vi "CycleHistoryTable.vi"(5 "Low Level Tries":u8=5, 7 "Error In":errorcluster, 8 "Cycle History ERD":T1={"ERD Number"=57629, "Data Type"=enum."string"} {"ERD Number" format="%.0x"}, 9 "GEA Inputs":T3={"Source"=228, "Destination"=36} {"Destination" format="%.0x"; "Source" format="%.0x"}, 10 "GEA2 Reference In":refnum<k24>) -> (0 "Error Out":errorcluster, 1 "String Array Out":string[](array[string]), 2 "Cluster Data Out":T4, 3 "GEA2 Reference Out":refnum<k24>)   [LabVIEW 2016]
uses:
  type defs/CycleHistoryControl.ctl
  Q:/Common/DLLs/GEA3/GeaCommunication.dll
  Common/DLLs/GEA3/GeaCommunication.dll
  Common/LabVIEW GEA2 Toolkit/LabVIEW_GEA2_Toolkit.lvlibp/type defs/Source_Destination.ctl
  Common/LabVIEW GEA2 Toolkit/LabVIEW_GEA2_Toolkit.lvlibp/type defs/ERD Read Data In.ctl
  Common/LabVIEW GEA2 Toolkit/LabVIEW_GEA2_Toolkit.lvlibp/type defs/Data Type.ctl
  Common/LabVIEW GEA2 Toolkit/LabVIEW_GEA2_Toolkit.lvlibp
panel:
  # "**Note: Two unused bytes at end**"
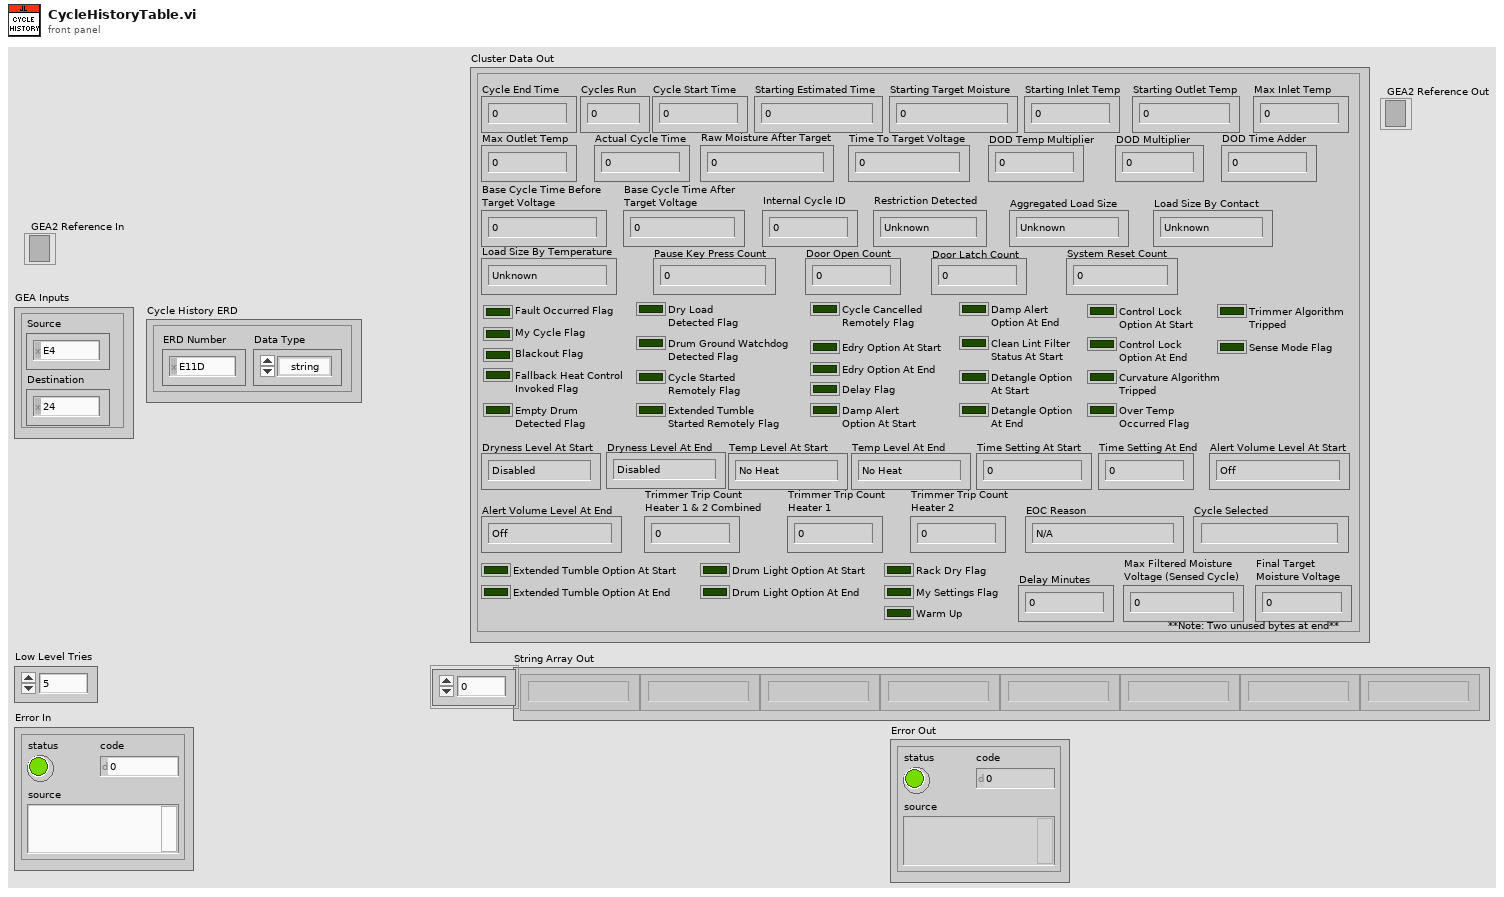
[diagram p1: front panel]
types:
  T1 = typedef "LabVIEW_GEA2_Toolkit.lvlibp/ERD Read Data In.ctl" = cluster{"ERD Number":u16, "Data Type":T2}
  T2 = typedef "LabVIEW_GEA2_Toolkit.lvlibp/Data Type.ctl" = enum16{"string", "boolean", "uint8_t", "uint16_t", "uint32_t", "uint64_t", "int8_t", "int16_t", "int32_t", "int64_t"}
  T3 = typedef "LabVIEW_GEA2_Toolkit.lvlibp/Source_Destination.ctl" = cluster{"Source":u8, "Destination":u8}
  T4 = typedef "CycleHistoryControl.ctl" = cluster{"Cycle End Time":u32, "Cycles Run":u32, "Cycle Start Time":u32, "Starting Estimated Time":u16, "Starting Target Moisture":u16, "Starting Inlet Temp":u16, "Starting Outlet Temp":u16, "Max Inlet Temp":u16, "Max Outlet Temp":u16, "Dryness Level At Start":enum8{"Disabled", "Damp", "Less Dry", "Dry", "More Dry", "Extra Dry"}, "Dryness Level At End":enum8{"Disabled", "Damp", "Less Dry", "Dry", "More Dry", "Extra Dry"}, "Temp Level At Start":enum8{"No Heat", "Extra Low", "Low", "Medium", "High"}, "Temp Level At End":enum8{"No Heat", "Extra Low", "Low", "Medium", "High"}, "Time Setting At Start":u8, "Time Setting At End":u8, "Trimmer Trip Count\nHeater 1 & 2 Combined":u8, "Trimmer Trip Count\nHeater 1":u8, "Trimmer Trip Count\nHeater 2":u8, "EOC Reason":enum16{"N/A", "Empty Drum", "Dry Load", "Cool Down Paused", "Extended Tumble Paused", "Knob Change", "Power Key", "Normal", "Event Sequence Communication Issue"}, "Cycle Selected":string, "Actual Cycle Time":u16, "Raw Moisture After Target":u16, "Time To Target Voltage":u16, "DOD Temp Multiplier":u16, "DOD Multiplier":u8, "DOD Time Adder":u8, "Base Cycle Time Before\nTarget Voltage":u8, "Base Cycle Time After\nTarget Voltage":u8, "Internal Cycle ID":u8, "Restriction Detected":enum8{"Unknown", "Small", "Large"}, "Aggregated Load Size":enum8{"Unknown", "Small", "Large"}, "Load Size By Contact":enum8{"Unknown", "Small", "Large"}, "Load Size By Temperature":enum8{"Unknown", "Small", "Large"}, "Pause Key Press Count":u8, "Door Open Count":u8, "Door Latch Count":u8, "System Reset Count":u8, "Fault Occurred Flag":bool, "My Cycle Flag":bool, "Blackout Flag":bool, "Fallback Heat Control\nInvoked Flag":bool, "Empty Drum \nDetected Flag":bool, "Dry Load \nDetected Flag":bool, "Drum Ground Watchdog\nDetected Flag":bool, "Cycle Started\nRemotely Flag":bool, "Extended Tumble\nStarted Remotely Flag":bool, "Cycle Cancelled\nRemotely Flag":bool, "Edry Option At Start":bool, "Edry Option At End":bool, "Delay Flag":bool, "Damp Alert\nOption At Start":bool, "Damp Alert\nOption At End":bool, "Clean Lint Filter\nStatus At Start":bool, "Detangle Option\nAt Start":bool, "Detangle Option\nAt End":bool, "Control Lock\nOption At Start":bool, "Control Lock\nOption At End":bool, "Curvature Algorithm\nTripped":bool, "Over Temp\nOccurred Flag":bool, "Trimmer Algorithm\nTripped":bool, "Sense Mode Flag":bool, "Extended Tumble Option At Start":bool, "Extended Tumble Option At End":bool, "Drum Light Option At Start":bool, "Drum Light Option At End":bool, "Rack Dry Flag":bool, "My Settings Flag":bool, "Warm Up":bool, "Delay Minutes":u16, "Alert Volume Level At Start":enum8{"Off", "Low", "Medium", "High"}, "Alert Volume Level At End":enum8{"Off", "Low", "Medium", "High"}, "Max Filtered Moisture\nVoltage (Sensed Cycle)":u16, "Final Target\nMoisture Voltage":u16}
  T5 = enum8{"Disabled", "Damp", "Less Dry", "Dry", "More Dry", "Extra Dry"}
  T6 = enum8{"No Heat", "Extra Low", "Low", "Medium", "High"}
  T7 = enum16{"N/A", "Empty Drum", "Dry Load", "Cool Down Paused", "Extended Tumble Paused", "Knob Change", "Power Key", "Normal", "Event Sequence Communication Issue"}
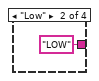
[diagram p4: hidden frame]
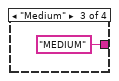
[diagram p5: hidden frame]
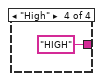
[diagram p6: hidden frame]
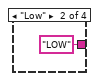
[diagram p7: hidden frame]
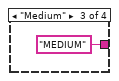
[diagram p8: hidden frame]
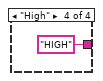
[diagram p9: hidden frame]
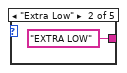
[diagram p10: hidden frame]
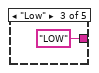
[diagram p11: hidden frame]
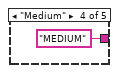
[diagram p12: hidden frame]
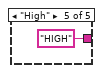
[diagram p13: hidden frame]
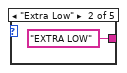
[diagram p14: hidden frame]
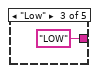
[diagram p15: hidden frame]
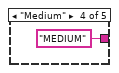
[diagram p16: hidden frame]
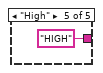
[diagram p17: hidden frame]
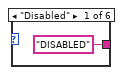
[diagram p18: hidden frame]
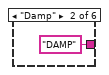
[diagram p19: hidden frame]
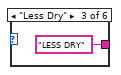
[diagram p20: hidden frame]
diagram:
  w24 = 3 ("offset (0)")
  w199 = 0 ("offset (0)")
  # "Final Target\nMoisture Voltage"
  # "Max Filtered Mosture\nDuring a Sensed Cycle"
  # "Take in a 1D array of ERD data\nfrom another VI & index that array\nto pull out the data. \n\nWe will parse this data in the next step..."
  # "Build a 1D array of strings \ncontaining all clustered data"
  # "Unbundle clustered data,\nthen format into string to\nobtain all clustered data as \none singlular string"
  # "Output clustered data\n& move to unbundle\ndata to format into \none string"
  # "Parse the data byte by byte...\nadd 3 each time since  each byte's\nlength is 2 numbers + 1 space character.\n\nThis number we are adding takes a subset\nof the data string to know which byte\nlocation we want to pull data from each time."
  # "Can try to use 'format into string' VI to\nsimplify this part, but should work as is."
  # "Alert Volume Level At End"
  # "Alert Volume Level At Start"
  # "Warm Up"
  # "Delay Minutes"
  # "=====CLUSTER ARRAY====="
  # "=====STRING ARRAY====="
  # "My Settings Flag"
  # "Rack Dry Flag"
  # "Drum Light Option At End"
  # "Drum Light Option At Start"
  # "Extended Tumble Option At End"
  # "Extended Tumble Option At Start"
  # "Boolean Byte #4"
  # "Cycle Selected"
  # "EOC Reason"
  # "Trimmer Trip Count Heater 2"
  # "Trimmer Trip Count Heater 1"
  # "Trimmer Trip Count\n Heater 1 & 2 Combined"
  # "Time Setting At End"
  # "Time Setting At Start"
  # "Temp Level At End"
  # "Temp Level At Start"
  # "Dryness Level At End"
  # "Dryness Level At Start"
  # "Sense Mode Flag"
  # "Trimmer Algorithm Tripped"
  # "Over Temperature Occurred Flag"
  # "Curvature Algorithm Tripped"
  # "Control Lock Option At End"
  # "Control Lock Option At Start"
  # "Detangle Option At End"
  # "Detangle Option At Start"
  # "Boolean Byte #3"
  # "Clean Lint Filter Status At Start"
  # "Damp Alert Option At End"
  # "Damp Alert Option At Start"
  # "Edry Option At End"
  # "Edry Option At Start"
  # "Cycle Cancelled Remotely Flag"
  # "Extended Tumble Started Remotely Flag"
  # "Cycle Started Remotely Flag"
  # "Boolean Byte #2"
  # "Drum Ground Watchdog Detected Flag"
  # "Dry Load Detected Flag"
  # "Empty Drum Detected Flag"
  # "Fallback Heat Control Invoked Flag"
  # "Blackout Flag"
  # "My Cycle Flag"
  # "Delay Flag"
  # "Fault Occurred Flag"
  # "Boolean Byte #1"
  # "Door Latch Count"
  # "System Reset Count"
  # "Door Open Count"
  # "Pause Key Press Count"
  # "Load Size By Temperature"
  # "Load Size By Contact"
  # "Aggregated Load Size"
  # "Restriction Detected"
  # "Internal Cycle ID"
  # "Base Cycle Time After\nTarget Voltage"
  # "Base Cycle Time Before\nTarget Voltage"
  # "DOD Time Adder"
  # "DOD Multiplier"
  # "DOD Temp Multiplier"
  # "Time To Target Voltage"
  # "Raw Moisture After Target"
  # "Actual Cycle Time"
  # "Max Outlet Temp"
  # "Max Inlet Temp"
  # "Starting Outlet Temp"
  # "Starting Inlet Temp"
  # "Starting Target Moisture"
  # "Starting Estimated Time"
  # "Cycle Start Time"
  # "Cycles Run"
  # "Cycle End Time"
  n1 = Not A Number/Path/Refnum?(number/path/refnum="GEA2 Reference In") -> (NaN/Path/Refnum?=w15:bool)
  n2 = case shown="True" w15 {
    tunnel: "GEA Inputs" -> [_ w635]
    tunnel: "Error In" -> [w630 w634]
    tunnel: [w630 w633] -> w8
    tunnel: [w629 w632] -> w13
    tunnel: "GEA2 Reference In" -> [w629 _]
    frame False {
    }
    frame True {
      n3 = Unbundle By Name(w635) -> ("Source"=w631:u8)
      n4 = call "GEA2 Initialize.vi"("Source Address"=w631, "error in"=w634) -> ("GEA2 Reference Out"=w632:refnum<k24>, "error out"=w633:errorcluster)  [unwired: 11 in, 1 out]
    }
  }
  n5 = Build Array("Cycle History ERD") -> (w4:T1[])
  n6 = call "GEA2 Read ERD.vi"("GEA2 Reference In"=w13, "GEA Inputs"="GEA Inputs", "Read ERD List"=w4, "Error In"=w8, "Low Level Tries"="Low Level Tries") -> ("GEA2 Reference Out"=w11:refnum<k24>, "Raw Data Out"=w9:string, "Error Out"=w10:errorcluster)  [unwired: 7 in, 1 out]
  n7 = case shown="True" w15 {
    tunnel: [w636 w640] -> w16
    tunnel: [w637 _] -> w14
    tunnel: w11 -> [w637 w638]
    tunnel: w10 -> [w636 w639]
    frame False {
    }
    frame True {
      n8 = call "GEA2 Stop.vi"("GEA2 Reference In"=w638, "Error In"=w639) -> ("Error Out"=w640:errorcluster)  [unwired: 13 in]
    }
  }
  "Error Out" <- w16
  "GEA2 Reference Out" <- w14
  n9 = String Subset(string=w9, offset (0)=28) -> (substring=w2:string)  [unwired: 1 in]
  n10 = call "String Remove All Spaces.vi"("Input String"=w2) -> ("Spaces Removed"=w1:string)  [unwired: 13 in, 1 out]
  n11 = Add(x=w199, y=w24) -> (x+y=w198:i32)
  n12 = Add(x=w198, y=w24) -> (x+y=w197:i32)
  n13 = Add(x=w197, y=w24) -> (x+y=w196:i32)
  n14 = Add(x=w196, y=w24) -> (x+y=w195:i32)
  n15 = Add(x=w195, y=w24) -> (x+y=w194:i32)
  n16 = Add(x=w194, y=w24) -> (x+y=w193:i32)
  n17 = Add(x=w193, y=w24) -> (x+y=w192:i32)
  n18 = Add(x=w192, y=w24) -> (x+y=w191:i32)
  n19 = Add(x=w191, y=w24) -> (x+y=w190:i32)
  n20 = Add(x=w190, y=w24) -> (x+y=w189:i32)
  n21 = Add(x=w189, y=w24) -> (x+y=w188:i32)
  n22 = Add(x=w188, y=w24) -> (x+y=w187:i32)
  n23 = Add(x=w187, y=w24) -> (x+y=w186:i32)
  n24 = Add(x=w186, y=w24) -> (x+y=w185:i32)
  n25 = Add(x=w185, y=w24) -> (x+y=w184:i32)
  n26 = Add(x=w184, y=w24) -> (x+y=w183:i32)
  n27 = Add(x=w183, y=w24) -> (x+y=w182:i32)
  n28 = Add(x=w182, y=w24) -> (x+y=w181:i32)
  n29 = Add(x=w181, y=w24) -> (x+y=w180:i32)
  n30 = Add(x=w180, y=w24) -> (x+y=w179:i32)
  n31 = Add(x=w179, y=w24) -> (x+y=w178:i32)
  n32 = Add(x=w178, y=w24) -> (x+y=w177:i32)
  n33 = Add(x=w177, y=w24) -> (x+y=w176:i32)
  n34 = Add(x=w176, y=w24) -> (x+y=w175:i32)
  n35 = Add(x=w175, y=w24) -> (x+y=w174:i32)
  n36 = Add(x=w174, y=w24) -> (x+y=w173:i32)
  n37 = Add(x=w173, y=w24) -> (x+y=w172:i32)
  n38 = Add(x=w172, y=w24) -> (x+y=w171:i32)
  n39 = Add(x=w171, y=w24) -> (x+y=w170:i32)
  n40 = Add(x=w170, y=w24) -> (x+y=w169:i32)
  n41 = Add(x=w169, y=w24) -> (x+y=w160:i32)
  n42 = Add(x=w160, y=w24) -> (x+y=w158:i32)
  n43 = Add(x=w158, y=w24) -> (x+y=w157:i32)
  n44 = Add(x=w157, y=w24) -> (x+y=w150:i32)
  n45 = Add(x=w150, y=w24) -> (x+y=w148:i32)
  n46 = Add(x=w148, y=w24) -> (x+y=w146:i32)
  n47 = Add(x=w146, y=w24) -> (x+y=w144:i32)
  n48 = Add(x=w144, y=w24) -> (x+y=w142:i32)
  n49 = Add(x=w142, y=w24) -> (x+y=w140:i32)
  n50 = Add(x=w140, y=w24) -> (x+y=w137:i32)
  n51 = Add(x=w137, y=w24) -> (x+y=w136:i32)
  n52 = Add(x=w136, y=w24) -> (x+y=w134:i32)
  n53 = Add(x=w134, y=w24) -> (x+y=w132:i32)
  n54 = Add(x=w132, y=w24) -> (x+y=w130:i32)
  n55 = Add(x=w130, y=w24) -> (x+y=w128:i32)
  n56 = Add(x=w128, y=w24) -> (x+y=w126:i32)
  n57 = Add(x=w126, y=w24) -> (x+y=w124:i32)
  n58 = Add(x=w124, y=w24) -> (x+y=w122:i32)
  n59 = Add(x=w122, y=w24) -> (x+y=w120:i32)
  n60 = Add(x=w120, y=w24) -> (x+y=w118:i32)
  n61 = Add(x=w118, y=w24) -> (x+y=w116:i32)
  n62 = Add(x=w116, y=w24) -> (x+y=w114:i32)
  n63 = Add(x=w114, y=w24) -> (x+y=w112:i32)
  n64 = Add(x=w112, y=w24) -> (x+y=w110:i32)
  n65 = Add(x=w110, y=w24) -> (x+y=w76:i32)
  n66 = Add(x=w76, y=w24) -> (x+y=w78:i32)
  n67 = Add(x=w78, y=w24) -> (x+y=w73:i32)
  n68 = Add(x=w73, y=w24) -> (x+y=w107:i32)
  n69 = Add(x=w107, y=w24) -> (x+y=w105:i32)
  n70 = Add(x=w105, y=w24) -> (x+y=w103:i32)
  n71 = Add(x=w103, y=w24) -> (x+y=w101:i32)
  n72 = Add(x=w101, y=w24) -> (x+y=w94:i32)
  n73 = Add(x=w94, y=w24) -> (x+y=w92:i32)
  n74 = Add(x=w92, y=w24) -> (x+y=w90:i32)
  n75 = Add(x=w90, y=w24) -> (x+y=w41:i32)
  n76 = Add(x=w41, y=w24) -> (x+y=w38:i32)
  n77 = Add(x=w38, y=w24) -> (x+y=w25:i32)
  n78 = Add(x=w25, y=w24) -> (x+y=w31:i32)
  n79 = Add(x=w31, y=w24) -> (x+y=w30:i32)
  n80 = String Subset(string=w1, offset (0)=w198, length (rest)=2 ("length (rest)")) -> (substring=w622:string)
  n81 = String Subset(string=w1, offset (0)=w194, length (rest)=2 ("length (rest)")) -> (substring=w613:string)
  n82 = String Subset(string=w1, offset (0)=w199, length (rest)=2 ("length (rest)")) -> (substring=w623:string)
  n83 = String Subset(string=w1, offset (0)=w195, length (rest)=2 ("length (rest)")) -> (substring=w614:string)
  n84 = String Subset(string=w1, offset (0)=w197, length (rest)=2 ("length (rest)")) -> (substring=w621:string)
  n85 = String Subset(string=w1, offset (0)=w193, length (rest)=2 ("length (rest)")) -> (substring=w612:string)
  n86 = String Subset(string=w1, offset (0)=w196, length (rest)=2 ("length (rest)")) -> (substring=w620:string)
  n87 = String Subset(string=w1, offset (0)=w192, length (rest)=2 ("length (rest)")) -> (substring=w611:string)
  n88 = String Subset(string=w1, offset (0)=w190, length (rest)=2 ("length (rest)")) -> (substring=w602:string)
  n89 = String Subset(string=w1, offset (0)=w184, length (rest)=2 ("length (rest)")) -> (substring=w589:string)
  n90 = String Subset(string=w1, offset (0)=w183, length (rest)=2 ("length (rest)")) -> (substring=w583:string)
  n91 = String Subset(string=w1, offset (0)=w191, length (rest)=2 ("length (rest)")) -> (substring=w603:string)
  n92 = String Subset(string=w1, offset (0)=w185, length (rest)=2 ("length (rest)")) -> (substring=w590:string)
  n93 = String Subset(string=w1, offset (0)=w182, length (rest)=2 ("length (rest)")) -> (substring=w582:string)
  n94 = String Subset(string=w1, offset (0)=w186, length (rest)=2 ("length (rest)")) -> (substring=w595:string)
  n95 = String Subset(string=w1, offset (0)=w181, length (rest)=2 ("length (rest)")) -> (substring=w576:string)
  n96 = String Subset(string=w1, offset (0)=w187, length (rest)=2 ("length (rest)")) -> (substring=w596:string)
  n97 = String Subset(string=w1, offset (0)=w180, length (rest)=2 ("length (rest)")) -> (substring=w575:string)
  n98 = String Subset(string=w1, offset (0)=w189, length (rest)=2 ("length (rest)")) -> (substring=w601:string)
  n99 = String Subset(string=w1, offset (0)=w188, length (rest)=2 ("length (rest)")) -> (substring=w600:string)
  n100 = String Subset(string=w1, offset (0)=w179, length (rest)=2 ("length (rest)")) -> (substring=w569:string)
  n101 = String Subset(string=w1, offset (0)=w178, length (rest)=2 ("length (rest)")) -> (substring=w568:string)
  n102 = String Subset(string=w1, offset (0)=w177, length (rest)=2 ("length (rest)")) -> (substring=w563:string)
  n103 = String Subset(string=w1, offset (0)=w176, length (rest)=2 ("length (rest)")) -> (substring=w562:string)
  n104 = String Subset(string=w1, offset (0)=w92, length (rest)=2 ("length (rest)")) -> (substring=w342:string)
  n105 = String Subset(string=w1, offset (0)=w175, length (rest)=2 ("length (rest)")) -> (substring=w555:string)
  n106 = String Subset(string=w1, offset (0)=w103, length (rest)=2 ("length (rest)")) -> (substring=w355:string)
  n107 = String Subset(string=w1, offset (0)=w94, length (rest)=2 ("length (rest)")) -> (substring=w346:string)
  n108 = String Subset(string=w1, offset (0)=w174, length (rest)=2 ("length (rest)")) -> (substring=w554:string)
  n109 = String Subset(string=w1, offset (0)=w76, length (rest)=2 ("length (rest)")) -> (substring=w362:string)
  n110 = String Subset(string=w1, offset (0)=w107, length (rest)=2 ("length (rest)")) -> (substring=w357:string)
  n111 = String Subset(string=w1, offset (0)=w105, length (rest)=2 ("length (rest)")) -> (substring=w356:string)
  n112 = String Subset(string=w1, offset (0)=w101, length (rest)=2 ("length (rest)")) -> (substring=w351:string)
  n113 = String Subset(string=w1, offset (0)=w173, length (rest)=2 ("length (rest)")) -> (substring=w549:string)
  n114 = String Subset(string=w1, offset (0)=w144, length (rest)=2 ("length (rest)")) -> (substring=w527:string)
  n115 = String Subset(string=w1, offset (0)=w110, length (rest)=2 ("length (rest)")) -> (substring=w363:string)
  n116 = String Subset(string=w1, offset (0)=w172, length (rest)=2 ("length (rest)")) -> (substring=w548:string)
  n117 = String Subset(string=w1, offset (0)=w146, length (rest)=2 ("length (rest)")) -> (substring=w529:string)
  n118 = String Subset(string=w1, offset (0)=w112, length (rest)=2 ("length (rest)")) -> (substring=w367:string)
  n119 = String Subset(string=w1, offset (0)=w142, length (rest)=2 ("length (rest)")) -> (substring=w523:string)
  n120 = String Subset(string=w1, offset (0)=w116, length (rest)=2 ("length (rest)")) -> (substring=w369:string)
  n121 = String Subset(string=w1, offset (0)=w114, length (rest)=2 ("length (rest)")) -> (substring=w368:string)
  n122 = String Subset(string=w1, offset (0)=w31, length (rest)=2 ("length (rest)")) -> (substring=w29:string)
  n123 = String Subset(string=w1, offset (0)=w148, length (rest)=2 ("length (rest)")) -> (substring=w154:string)
  n124 = String Subset(string=w1, offset (0)=w134, length (rest)=2 ("length (rest)")) -> (substring=w515:string)
  n125 = String Subset(string=w1, offset (0)=w118, length (rest)=2 ("length (rest)")) -> (substring=w371:string)
  n126 = String Subset(string=w1, offset (0)=w90, length (rest)=2 ("length (rest)")) -> (substring=w99:string)
  n127 = String Subset(string=w1, offset (0)=w41, length (rest)=2 ("length (rest)")) -> (substring=w98:string)
  n128 = String Subset(string=w1, offset (0)=w30, length (rest)=2 ("length (rest)")) -> (substring=w28:string)
  n129 = String Subset(string=w1, offset (0)=w171, length (rest)=2 ("length (rest)")) -> (substring=w541:string)
  n130 = String Subset(string=w1, offset (0)=w157, length (rest)=2 ("length (rest)")) -> (substring=w165:string)
  n131 = String Subset(string=w1, offset (0)=w170, length (rest)=2 ("length (rest)")) -> (substring=w540:string)
  n132 = String Subset(string=w1, offset (0)=w150, length (rest)=2 ("length (rest)")) -> (substring=w155:string)
  n133 = String Subset(string=w1, offset (0)=w132, length (rest)=2 ("length (rest)")) -> (substring=w512:string)
  n134 = String Subset(string=w1, offset (0)=w169, length (rest)=2 ("length (rest)")) -> (substring=w535:string)
  n135 = String Subset(string=w1, offset (0)=w158, length (rest)=2 ("length (rest)")) -> (substring=w166:string)
  n136 = String Subset(string=w1, offset (0)=w137, length (rest)=2 ("length (rest)")) -> (substring=w518:string)
  n137 = String Subset(string=w1, offset (0)=w136, length (rest)=2 ("length (rest)")) -> (substring=w516:string)
  n138 = String Subset(string=w1, offset (0)=w130, length (rest)=2 ("length (rest)")) -> (substring=w511:string)
  n139 = String Subset(string=w1, offset (0)=w120, length (rest)=2 ("length (rest)")) -> (substring=w430:string)
  n140 = String Subset(string=w1, offset (0)=w160, length (rest)=2 ("length (rest)")) -> (substring=w534:string)
  n141 = String Subset(string=w1, offset (0)=w128, length (rest)=2 ("length (rest)")) -> (substring=w510:string)
  n142 = String Subset(string=w1, offset (0)=w126, length (rest)=2 ("length (rest)")) -> (substring=w509:string)
  n143 = String Subset(string=w1, offset (0)=w140, length (rest)=2 ("length (rest)")) -> (substring=w520:string)
  n144 = String Subset(string=w1, offset (0)=w122, length (rest)=2 ("length (rest)")) -> (substring=w465:string)
  n145 = String Subset(string=w1, offset (0)=w124, length (rest)=2 ("length (rest)")) -> (substring=w500:string)
  n146 = String Subset(string=w1, offset (0)=w73, length (rest)=2 ("length (rest)")) -> (substring=w80:string)
  n147 = String Subset(string=w1, offset (0)=w38, length (rest)=2 ("length (rest)")) -> (substring=w37:string)
  n148 = String Subset(string=w1, offset (0)=w78, length (rest)=2 ("length (rest)")) -> (substring=w81:string)
  n149 = String Subset(string=w1, offset (0)=w25, length (rest)=2 ("length (rest)")) -> (substring=w36:string)
  n150 = Hexadecimal String To Number(string=w342) -> (number=w341:u32)  [unwired: 2 in, 1 out]
  n151 = Concatenate Strings(w623, w622, w621, w620) -> (w619:string)
  n152 = Concatenate Strings(w614, w613, w612, w611) -> (w610:string)
  n153 = Concatenate Strings(w590, w589) -> (w588:string)
  n154 = Concatenate Strings(w603, w602, w601, w600) -> (w599:string)
  n155 = Concatenate Strings(w596, w595) -> (w594:string)
  n156 = Hexadecimal String To Number(string=w430) -> (number=w429:u32)  [unwired: 2 in, 1 out]
  n157 = Hexadecimal String To Number(string=w465) -> (number=w464:u32)  [unwired: 2 in, 1 out]
  n158 = Concatenate Strings(w583, w582) -> (w580:string)
  n159 = Hexadecimal String To Number(string=w500) -> (number=w499:u32)  [unwired: 2 in, 1 out]
  n160 = Concatenate Strings(w576, w575) -> (w573:string)
  n161 = Concatenate Strings(w569, w568) -> (w566:string)
  n162 = Concatenate Strings(w563, w562) -> (w560:string)
  n163 = Concatenate Strings(w555, w554) -> (w552:string)
  n164 = Concatenate Strings(w29, w28) -> (w27:string)
  n165 = Concatenate Strings(w549, w548) -> (w546:string)
  n166 = Concatenate Strings(w99, w98) -> (w96:string)
  n167 = Hexadecimal String To Number(string=w355) -> (number=w352:u32)  [unwired: 2 in, 1 out]
  n168 = Hexadecimal String To Number(string=w346) -> (number=w345:u32)  [unwired: 2 in, 1 out]
  n169 = Hexadecimal String To Number(string=w362) -> (number=w360:u32)  [unwired: 2 in, 1 out]
  n170 = Hexadecimal String To Number(string=w357) -> (number=w354:u32)  [unwired: 2 in, 1 out]
  n171 = Hexadecimal String To Number(string=w356) -> (number=w353:u32)  [unwired: 2 in, 1 out]
  n172 = Hexadecimal String To Number(string=w351) -> (number=w347:u32)  [unwired: 2 in, 1 out]
  n173 = Concatenate Strings(w541, w540) -> (w538:string)
  n174 = Hexadecimal String To Number(string=w527) -> (number=w526:u32)  [unwired: 2 in, 1 out]
  n175 = Hexadecimal String To Number(string=w363) -> (number=w361:u32)  [unwired: 2 in, 1 out]
  n176 = Hexadecimal String To Number(string=w529) -> (number=w528:u32)  [unwired: 2 in, 1 out]
  n177 = Hexadecimal String To Number(string=w367) -> (number=w364:u32)  [unwired: 2 in, 1 out]
  n178 = Concatenate Strings(w535, w534) -> (w532:string)
  n179 = Hexadecimal String To Number(string=w523) -> (number=w522:u32)  [unwired: 2 in, 1 out]
  n180 = Hexadecimal String To Number(string=w369) -> (number=w366:u32)  [unwired: 2 in, 1 out]
  n181 = Hexadecimal String To Number(string=w368) -> (number=w365:u32)  [unwired: 2 in, 1 out]
  n182 = Hexadecimal String To Number(string=w515) -> (number=w513:u32)  [unwired: 2 in, 1 out]
  n183 = Hexadecimal String To Number(string=w371) -> (number=w370:u32)  [unwired: 2 in, 1 out]
  n184 = Number To Boolean Array(number=w341) -> (Boolean array=w83:bool[])
  n185 = Concatenate Strings(w37, w36) -> (w35:string)
  n186 = Concatenate Strings(w166, w165) -> (w164:string)
  n187 = Concatenate Strings(w155, w154) -> (w153:string)
  n188 = Hexadecimal String To Number(string=w512) -> (number=w508:u32)  [unwired: 2 in, 1 out]
  n189 = Hexadecimal String To Number(string=w518) -> (number=w517:u32)  [unwired: 2 in, 1 out]
  n190 = Hexadecimal String To Number(string=w516) -> (number=w514:u32)  [unwired: 2 in, 1 out]
  n191 = Hexadecimal String To Number(string=w511) -> (number=w506:u32)  [unwired: 2 in, 1 out]
  n192 = Hexadecimal String To Number(string=w510) -> (number=w504:u32)  [unwired: 2 in, 1 out]
  n193 = Hexadecimal String To Number(string=w509) -> (number=w503:u32)  [unwired: 2 in, 1 out]
  n194 = Hexadecimal String To Number(string=w520) -> (number=w519:u32)  [unwired: 2 in, 1 out]
  n195 = Hexadecimal String To Number(string=w80) -> (number=w74:u32)  [unwired: 2 in, 1 out]
  n196 = Number To Boolean Array(number=w429) -> (Boolean array=w396:bool[])
  n197 = Hexadecimal String To Number(string=w81) -> (number=w75:u32)  [unwired: 2 in, 1 out]
  n198 = Number To Boolean Array(number=w464) -> (Boolean array=w431:bool[])
  n199 = Number To Boolean Array(number=w499) -> (Boolean array=w466:bool[])
  n200 = Hexadecimal String To Number(string=w619) -> (number=w609:u32)  [unwired: 2 in, 1 out]
  n201 = Hexadecimal String To Number(string=w610) -> (number=w608:u32)  [unwired: 2 in, 1 out]
  n202 = Hexadecimal String To Number(string=w588) -> (number=w587:u32)  [unwired: 2 in, 1 out]
  n203 = Hexadecimal String To Number(string=w594) -> (number=w593:u32)  [unwired: 2 in, 1 out]
  n204 = Hexadecimal String To Number(string=w599) -> (number=w598:u32)  [unwired: 2 in, 1 out]
  n205 = Hexadecimal String To Number(string=w580) -> (number=w581:u32)  [unwired: 2 in, 1 out]
  n206 = Hexadecimal String To Number(string=w573) -> (number=w574:u32)  [unwired: 2 in, 1 out]
  n207 = To Unsigned Byte Integer(number=w345) -> (unsigned 8bit integer=w344:u8)
  n208 = To Unsigned Byte Integer(number=w361) -> (unsigned 8bit integer=w359:u8)
  n209 = To Unsigned Byte Integer(number=w360) -> (unsigned 8bit integer=w358:u8)
  n210 = To Unsigned Byte Integer(number=w354) -> (unsigned 8bit integer=w350:u8)
  n211 = Hexadecimal String To Number(string=w566) -> (number=w567:u32)  [unwired: 2 in, 1 out]
  n212 = To Unsigned Byte Integer(number=w353) -> (unsigned 8bit integer=w349:u8)
  n213 = To Unsigned Byte Integer(number=w352) -> (unsigned 8bit integer=w348:u8)
  n214 = Hexadecimal String To Number(string=w27) -> (number=w26:u32)  [unwired: 2 in, 1 out]
  n215 = Hexadecimal String To Number(string=w560) -> (number=w561:u32)  [unwired: 2 in, 1 out]
  n216 = To Unsigned Byte Integer(number=w526) -> (unsigned 8bit integer=w524:u8)
  n217 = To Unsigned Byte Integer(number=w528) -> (unsigned 8bit integer=w525:u8)
  n218 = To Unsigned Byte Integer(number=w522) -> (unsigned 8bit integer=w521:u8)
  n219 = To Unsigned Byte Integer(number=w508) -> (unsigned 8bit integer=w507:u8)
  n220 = To Unsigned Byte Integer(number=w506) -> (unsigned 8bit integer=w505:u8)
  n221 = To Unsigned Byte Integer(number=w504) -> (unsigned 8bit integer=w502:u8)
  n222 = To Unsigned Byte Integer(number=w503) -> (unsigned 8bit integer=w501:u8)
  n223 = Hexadecimal String To Number(string=w96) -> (number=w97:u32)  [unwired: 2 in, 1 out]
  n224 = Hexadecimal String To Number(string=w552) -> (number=w553:u32)  [unwired: 2 in, 1 out]
  n225 = Hexadecimal String To Number(string=w35) -> (number=w34:u32)  [unwired: 2 in, 1 out]
  n226 = Hexadecimal String To Number(string=w546) -> (number=w547:u32)  [unwired: 2 in, 1 out]
  n227 = Hexadecimal String To Number(string=w153) -> (number=w152:u32)  [unwired: 2 in, 1 out]
  n228 = Hexadecimal String To Number(string=w538) -> (number=w539:u32)  [unwired: 2 in, 1 out]
  n229 = Hexadecimal String To Number(string=w164) -> (number=w168:u32)  [unwired: 2 in, 1 out]
  n230 = Hexadecimal String To Number(string=w532) -> (number=w533:u32)  [unwired: 2 in, 1 out]
  n231 = Array Subset(array=w83, index=5, length=1) -> (w317:bool[])
  n232 = Array Subset(array=w83, index=6, length=1) -> (w84:bool[])
  n233 = Array Subset(array=w83, index=0, length=1) -> (w325:bool[])
  n234 = Array Subset(array=w83, index=1, length=1) -> (w324:bool[])
  n235 = Array Subset(array=w83, index=2, length=1) -> (w323:bool[])
  n236 = Array Subset(array=w83, index=3, length=1) -> (w322:bool[])
  n237 = Array Subset(array=w83, index=4, length=1) -> (w321:bool[])
  n238 = To Unsigned Word Integer(number=w587) -> (unsigned 16bit integer=w586:u16)
  n239 = To Unsigned Word Integer(number=w593) -> (unsigned 16bit integer=w592:u16)
  n240 = Array Subset(array=w396, index=6, length=1) -> (w401:bool[])
  n241 = Array Subset(array=w396, index=5, length=1) -> (w405:bool[])
  n242 = Array Subset(array=w396, index=7, length=1) -> (w397:bool[])
  n243 = To Unsigned Word Integer(number=w581) -> (unsigned 16bit integer=w579:u16)
  n244 = Array Subset(array=w431, index=6, length=1) -> (w436:bool[])
  n245 = Array Subset(array=w396, index=0, length=1) -> (w413:bool[])
  n246 = Array Subset(array=w396, index=1, length=1) -> (w412:bool[])
  n247 = Array Subset(array=w396, index=2, length=1) -> (w411:bool[])
  n248 = Array Subset(array=w396, index=3, length=1) -> (w410:bool[])
  n249 = Array Subset(array=w396, index=4, length=1) -> (w409:bool[])
  n250 = To Unsigned Word Integer(number=w574) -> (unsigned 16bit integer=w572:u16)
  n251 = Array Subset(array=w466, index=6, length=1) -> (w471:bool[])
  n252 = Array Subset(array=w431, index=5, length=1) -> (w440:bool[])
  n253 = Array Subset(array=w431, index=7, length=1) -> (w432:bool[])
  n254 = Array Subset(array=w466, index=5, length=1) -> (w475:bool[])
  n255 = Array Subset(array=w466, index=7, length=1) -> (w467:bool[])
  n256 = Array Subset(array=w431, index=0, length=1) -> (w448:bool[])
  n257 = Array Subset(array=w431, index=1, length=1) -> (w447:bool[])
  n258 = Array Subset(array=w431, index=2, length=1) -> (w446:bool[])
  n259 = Array Subset(array=w431, index=3, length=1) -> (w445:bool[])
  n260 = Array Subset(array=w431, index=4, length=1) -> (w444:bool[])
  n261 = Array Subset(array=w466, index=0, length=1) -> (w483:bool[])
  n262 = Array Subset(array=w466, index=1, length=1) -> (w482:bool[])
  n263 = Array Subset(array=w466, index=2, length=1) -> (w481:bool[])
  n264 = Array Subset(array=w466, index=3, length=1) -> (w480:bool[])
  n265 = Array Subset(array=w466, index=4, length=1) -> (w479:bool[])
  n266 = To Unsigned Word Integer(number=w567) -> (unsigned 16bit integer=w559:u16)
  n267 = To Unsigned Word Integer(number=w561) -> (unsigned 16bit integer=w558:u16)
  n268 = To Unsigned Word Integer(number=w553) -> (unsigned 16bit integer=w545:u16)
  n269 = To Unsigned Word Integer(number=w26) -> (unsigned 16bit integer=w22:u16)
  n270 = To Unsigned Word Integer(number=w547) -> (unsigned 16bit integer=w544:u16)
  n271 = To Unsigned Word Integer(number=w539) -> (unsigned 16bit integer=w531:u16)
  n272 = To Unsigned Word Integer(number=w533) -> (unsigned 16bit integer=w530:u16)
  n273 = To Unsigned Word Integer(number=w168) -> (unsigned 16bit integer=w167:u16)
  n274 = To Unsigned Word Integer(number=w97) -> (unsigned 16bit integer=w95:u16)
  n275 = To Unsigned Word Integer(number=w34) -> (unsigned 16bit integer=w23:u16)
  n276 = To Unsigned Word Integer(number=w152) -> (unsigned 16bit integer=w151:u16)
  n277 = case shown="0, Default" w344 {
    tunnel: ["Not Defined" "Bulky Items" "Sanitize" "Towels/Sheets" "Mixed Load" "Jeans" "Delicates" "Cottons" "Easy Care" "Active Wear" "Timed Dry" "DeWrinkle" "Quick/Air Fluff" "Steam Refresh" "Steam Dewrinkle" "Speed Dry" "Mixed" "Quick dry" "Casuals" "Warm up" "Energy Saver"] -> w343
    frame 0, Default {
    }
    frame 4 {
    }
    frame 5 {
    }
    frame 6 {
    }
    frame 8 {
    }
    frame 11 {
    }
    frame 13 {
    }
    frame 128 {
    }
    frame 129 {
    }
    frame 130 {
    }
    frame 131 {
    }
    frame 132 {
    }
    frame 133 {
    }
    frame 134 {
    }
    frame 135 {
    }
    frame 136 {
    }
    frame 137 {
    }
    frame 138 {
    }
    frame 139 {
    }
    frame 140 {
    }
    frame 141 {
    }
  }
  n278 = Boolean Array To Number(Boolean array=w317) -> (number=w320:u32)
  n279 = Boolean Array To Number(Boolean array=w84) -> (number=w87:u32)
  n280 = Boolean Array To Number(Boolean array=w325) -> (number=w340:u32)
  n281 = Boolean Array To Number(Boolean array=w324) -> (number=w339:u32)
  n282 = Boolean Array To Number(Boolean array=w323) -> (number=w338:u32)
  n283 = Boolean Array To Number(Boolean array=w322) -> (number=w337:u32)
  n284 = Boolean Array To Number(Boolean array=w321) -> (number=w336:u32)
  n285 = Boolean Array To Number(Boolean array=w401) -> (number=w404:u32)
  n286 = Boolean Array To Number(Boolean array=w405) -> (number=w408:u32)
  n287 = Boolean Array To Number(Boolean array=w397) -> (number=w400:u32)
  n288 = Boolean Array To Number(Boolean array=w436) -> (number=w439:u32)
  n289 = Boolean Array To Number(Boolean array=w413) -> (number=w428:u32)
  n290 = Boolean Array To Number(Boolean array=w412) -> (number=w427:u32)
  n291 = Boolean Array To Number(Boolean array=w411) -> (number=w426:u32)
  n292 = Boolean Array To Number(Boolean array=w410) -> (number=w425:u32)
  n293 = Boolean Array To Number(Boolean array=w409) -> (number=w424:u32)
  n294 = Boolean Array To Number(Boolean array=w471) -> (number=w474:u32)
  n295 = Boolean Array To Number(Boolean array=w440) -> (number=w443:u32)
  n296 = Boolean Array To Number(Boolean array=w432) -> (number=w435:u32)
  n297 = Boolean Array To Number(Boolean array=w475) -> (number=w478:u32)
  n298 = Boolean Array To Number(Boolean array=w467) -> (number=w470:u32)
  n299 = Boolean Array To Number(Boolean array=w448) -> (number=w463:u32)
  n300 = Boolean Array To Number(Boolean array=w447) -> (number=w462:u32)
  n301 = Boolean Array To Number(Boolean array=w446) -> (number=w461:u32)
  n302 = Boolean Array To Number(Boolean array=w445) -> (number=w460:u32)
  n303 = Boolean Array To Number(Boolean array=w444) -> (number=w459:u32)
  n304 = Boolean Array To Number(Boolean array=w483) -> (number=w498:u32)
  n305 = Boolean Array To Number(Boolean array=w482) -> (number=w497:u32)
  n306 = Boolean Array To Number(Boolean array=w481) -> (number=w496:u32)
  n307 = Boolean Array To Number(Boolean array=w480) -> (number=w495:u32)
  n308 = Boolean Array To Number(Boolean array=w479) -> (number=w494:u32)
  n309 = case shown="0, Default" w320 {
    tunnel: [FALSE TRUE] -> w312
    tunnel: ["FALSE" "TRUE"] -> _
    frame 0, Default {
    }
    frame 1 {
    }
  }
  n310 = case shown="0, Default" w87 {
    tunnel: [FALSE TRUE] -> w82
    tunnel: ["FALSE" "TRUE"] -> _
    frame 0, Default {
    }
    frame 1 {
    }
  }
  n311 = case shown="0, Default" w340 {
    tunnel: [FALSE TRUE] -> w88
    tunnel: ["FALSE" "TRUE"] -> _
    frame 0, Default {
    }
    frame 1 {
    }
  }
  n312 = case shown="0, Default" w339 {
    tunnel: [FALSE TRUE] -> w316
    tunnel: ["FALSE" "TRUE"] -> _
    frame 0, Default {
    }
    frame 1 {
    }
  }
  n313 = case shown="0, Default" w338 {
    tunnel: [FALSE TRUE] -> w315
    tunnel: ["FALSE" "TRUE"] -> _
    frame 0, Default {
    }
    frame 1 {
    }
  }
  n314 = case shown="0, Default" w337 {
    tunnel: [FALSE TRUE] -> w314
    tunnel: ["FALSE" "TRUE"] -> _
    frame 0, Default {
    }
    frame 1 {
    }
  }
  n315 = case shown="0, Default" w336 {
    tunnel: [FALSE TRUE] -> w313
    tunnel: ["FALSE" "TRUE"] -> _
    frame 0, Default {
    }
    frame 1 {
    }
  }
  n316 = case shown="0, Default" w404 {
    tunnel: [FALSE TRUE] -> w373
    tunnel: ["FALSE" "TRUE"] -> _
    frame 0, Default {
    }
    frame 1 {
    }
  }
  n317 = case shown="0, Default" w408 {
    tunnel: [FALSE TRUE] -> w374
    tunnel: ["FALSE" "TRUE"] -> _
    frame 0, Default {
    }
    frame 1 {
    }
  }
  n318 = case shown="0, Default" w400 {
    tunnel: [FALSE TRUE] -> w372
    tunnel: ["FALSE" "TRUE"] -> _
    frame 0, Default {
    }
    frame 1 {
    }
  }
  n319 = case shown="0, Default" w439 {
    tunnel: [FALSE TRUE] -> w381
    tunnel: ["FALSE" "TRUE"] -> _
    frame 0, Default {
    }
    frame 1 {
    }
  }
  n320 = case shown="0, Default" w428 {
    tunnel: [FALSE TRUE] -> w379
    tunnel: ["FALSE" "TRUE"] -> _
    frame 0, Default {
    }
    frame 1 {
    }
  }
  n321 = case shown="0, Default" w427 {
    tunnel: [FALSE TRUE] -> w378
    tunnel: ["FALSE" "TRUE"] -> _
    frame 0, Default {
    }
    frame 1 {
    }
  }
  n322 = case shown="0, Default" w426 {
    tunnel: [FALSE TRUE] -> w377
    tunnel: ["FALSE" "TRUE"] -> _
    frame 0, Default {
    }
    frame 1 {
    }
  }
  n323 = case shown="0, Default" w425 {
    tunnel: [FALSE TRUE] -> w376
    tunnel: ["FALSE" "TRUE"] -> _
    frame 0, Default {
    }
    frame 1 {
    }
  }
  n324 = case shown="0, Default" w424 {
    tunnel: [FALSE TRUE] -> w375
    tunnel: ["FALSE" "TRUE"] -> _
    frame 0, Default {
    }
    frame 1 {
    }
  }
  n325 = case shown="0, Default" w474 {
    tunnel: [FALSE TRUE] -> w389
    tunnel: ["FALSE" "TRUE"] -> _
    frame 0, Default {
    }
    frame 1 {
    }
  }
  n326 = case shown="0, Default" w443 {
    tunnel: [FALSE TRUE] -> w382
    tunnel: ["FALSE" "TRUE"] -> _
    frame 0, Default {
    }
    frame 1 {
    }
  }
  n327 = case shown="0, Default" w435 {
    tunnel: [FALSE TRUE] -> w380
    tunnel: ["FALSE" "TRUE"] -> _
    frame 0, Default {
    }
    frame 1 {
    }
  }
  n328 = case shown="0, Default" w478 {
    tunnel: [FALSE TRUE] -> w390
    tunnel: ["FALSE" "TRUE"] -> _
    frame 0, Default {
    }
    frame 1 {
    }
  }
  n329 = case shown="0, Default" w470 {
    tunnel: [FALSE TRUE] -> w388
    tunnel: ["FALSE" "TRUE"] -> _
    frame 0, Default {
    }
    frame 1 {
    }
  }
  n330 = case shown="0, Default" w463 {
    tunnel: [FALSE TRUE] -> w387
    tunnel: ["FALSE" "TRUE"] -> _
    frame 0, Default {
    }
    frame 1 {
    }
  }
  n331 = case shown="0, Default" w462 {
    tunnel: [FALSE TRUE] -> w386
    tunnel: ["FALSE" "TRUE"] -> _
    frame 0, Default {
    }
    frame 1 {
    }
  }
  n332 = case shown="0, Default" w461 {
    tunnel: [FALSE TRUE] -> w385
    tunnel: ["FALSE" "TRUE"] -> _
    frame 0, Default {
    }
    frame 1 {
    }
  }
  n333 = case shown="0, Default" w460 {
    tunnel: [FALSE TRUE] -> w384
    tunnel: ["FALSE" "TRUE"] -> _
    frame 0, Default {
    }
    frame 1 {
    }
  }
  n334 = case shown="0, Default" w459 {
    tunnel: [FALSE TRUE] -> w383
    tunnel: ["FALSE" "TRUE"] -> _
    frame 0, Default {
    }
    frame 1 {
    }
  }
  n335 = case shown="0, Default" w498 {
    tunnel: [FALSE TRUE] -> w395
    tunnel: ["FALSE" "TRUE"] -> _
    frame 0, Default {
    }
    frame 1 {
    }
  }
  n336 = case shown="0, Default" w497 {
    tunnel: [FALSE TRUE] -> w394
    tunnel: ["FALSE" "TRUE"] -> _
    frame 0, Default {
    }
    frame 1 {
    }
  }
  n337 = case shown="0, Default" w496 {
    tunnel: [FALSE TRUE] -> w393
    tunnel: ["FALSE" "TRUE"] -> _
    frame 0, Default {
    }
    frame 1 {
    }
  }
  n338 = case shown="0, Default" w495 {
    tunnel: [FALSE TRUE] -> w392
    tunnel: ["FALSE" "TRUE"] -> _
    frame 0, Default {
    }
    frame 1 {
    }
  }
  n339 = case shown="0, Default" w494 {
    tunnel: [FALSE TRUE] -> w391
    tunnel: ["FALSE" "TRUE"] -> _
    frame 0, Default {
    }
    frame 1 {
    }
  }
  n340 = Bundle By Name(cluster=T4 {"Cycle End Time"=0, "Cycles Run"=0, "Cycle Start Time"=0, "Starting Estimated Time"=0, "Starting Target Moisture"=0, "Starting Inlet Temp"=0, "Starting Outlet Temp"=0, "Max Inlet Temp"=0, "Max Outlet Temp"=0, "Dryness Level At Start"=enum."Disabled", "Dryness Level At End"=enum."Disabled", "Temp Level At Start"=enum."No Heat", "Temp Level At End"=enum."No Heat", "Time Setting At Start"=0, "Time Setting At End"=0, "Trimmer Trip Count\nHeater 1 & 2 Combined"=0, "Trimmer Trip Count\nHeater 1"=0, "Trimmer Trip Count\nHeater 2"=0, "EOC Reason"=enum."N/A", "Cycle Selected"="", "Actual Cycle Time"=0, "Raw Moisture After Target"=0, "Time To Target Voltage"=0, "DOD Temp Multiplier"=0, "DOD Multiplier"=0, "DOD Time Adder"=0, "Base Cycle Time Before\nTarget Voltage"=0, "Base Cycle Time After\nTarget Voltage"=0, "Internal Cycle ID"=0, "Restriction Detected"=enum."Unknown", "Aggregated Load Size"=enum."Unknown", "Load Size By Contact"=enum."Unknown", "Load Size By Temperature"=enum."Unknown", "Pause Key Press Count"=0, "Door Open Count"=0, "Door Latch Count"=0, "System Reset Count"=0, "Fault Occurred Flag"=FALSE, "My Cycle Flag"=FALSE, "Blackout Flag"=FALSE, "Fallback Heat Control\nInvoked Flag"=FALSE, "Empty Drum \nDetected Flag"=FALSE, "Dry Load \nDetected Flag"=FALSE, "Drum Ground Watchdog\nDetected Flag"=FALSE, "Cycle Started\nRemotely Flag"=FALSE, "Extended Tumble\nStarted Remotely Flag"=FALSE, "Cycle Cancelled\nRemotely Flag"=FALSE, "Edry Option At Start"=FALSE, "Edry Option At End"=FALSE, "Delay Flag"=FALSE, "Damp Alert\nOption At Start"=FALSE, "Damp Alert\nOption At End"=FALSE, "Clean Lint Filter\nStatus At Start"=FALSE, "Detangle Option\nAt Start"=FALSE, "Detangle Option\nAt End"=FALSE, "Control Lock\nOption At Start"=FALSE, "Control Lock\nOption At End"=FALSE, "Curvature Algorithm\nTripped"=FALSE, "Over Temp\nOccurred Flag"=FALSE, "Trimmer Algorithm\nTripped"=FALSE, "Sense Mode Flag"=FALSE, "Extended Tumble Option At Start"=FALSE, "Extended Tumble Option At End"=FALSE, "Drum Light Option At Start"=FALSE, "Drum Light Option At End"=FALSE, "Rack Dry Flag"=FALSE, "My Settings Flag"=FALSE, "Warm Up"=FALSE, "Delay Minutes"=0, "Alert Volume Level At Start"=enum."Off", "Alert Volume Level At End"=enum."Off", "Max Filtered Moisture\nVoltage (Sensed Cycle)"=0, "Final Target\nMoisture Voltage"=0} ("Cycle History Cluster"), "Cycle End Time"=w609, "Cycles Run"=w608, "Cycle Start Time"=w598, "Starting Estimated Time"=w592, "Starting Target Moisture"=w586, "Starting Inlet Temp"=w579, "Starting Outlet Temp"=w572, "Max Inlet Temp"=w559, "Max Outlet Temp"=w558, "Actual Cycle Time"=w545, "Raw Moisture After Target"=w544, "Time To Target Voltage"=w531, "DOD Temp Multiplier"=w530, "DOD Multiplier"=w167, "DOD Time Adder"=w151, "Base Cycle Time Before\nTarget Voltage"=w525, "Base Cycle Time After\nTarget Voltage"=w524, "Internal Cycle ID"=w521, "Restriction Detected"=w519, "Aggregated Load Size"=w517, "Load Size By Contact"=w514, "Load Size By Temperature"=w513, "Pause Key Press Count"=w507, "Door Open Count"=w505, "Door Latch Count"=w502, "System Reset Count"=w501, "Fault Occurred Flag"=w395, "Delay Flag"=w394, "My Cycle Flag"=w393, "Blackout Flag"=w392, "Fallback Heat Control\nInvoked Flag"=w391, "Empty Drum \nDetected Flag"=w390, "Dry Load \nDetected Flag"=w389, "Drum Ground Watchdog\nDetected Flag"=w388, "Cycle Started\nRemotely Flag"=w387, "Extended Tumble\nStarted Remotely Flag"=w386, "Cycle Cancelled\nRemotely Flag"=w385, "Edry Option At Start"=w384, "Edry Option At End"=w383, "Damp Alert\nOption At Start"=w382, "Damp Alert\nOption At End"=w381, "Clean Lint Filter\nStatus At Start"=w380, "Detangle Option\nAt Start"=w379, "Detangle Option\nAt End"=w378, "Control Lock\nOption At Start"=w377, "Control Lock\nOption At End"=w376, "Curvature Algorithm\nTripped"=w375, "Over Temp\nOccurred Flag"=w374, "Trimmer Algorithm\nTripped"=w373, "Sense Mode Flag"=w372, "Dryness Level At Start"=w370, "Dryness Level At End"=w366, "Temp Level At Start"=w365, "Temp Level At End"=w364, "Time Setting At Start"=w359, "Time Setting At End"=w358, "Trimmer Trip Count\nHeater 1 & 2 Combined"=w350, "Trimmer Trip Count\nHeater 1"=w349, "Trimmer Trip Count\nHeater 2"=w348, "EOC Reason"=w347, "Cycle Selected"=w343, "Delay Minutes"=w95, "Extended Tumble Option At Start"=w88, "Extended Tumble Option At End"=w316, "Drum Light Option At Start"=w315, "Drum Light Option At End"=w314, "Rack Dry Flag"=w313, "My Settings Flag"=w312, "Warm Up"=w82, "Alert Volume Level At Start"=w75, "Alert Volume Level At End"=w74, "Max Filtered Moisture\nVoltage (Sensed Cycle)"=w23, "Final Target\nMoisture Voltage"=w22) -> (w628:T4)
  "Cluster Data Out" <- w628
  n341 = Unbundle By Name(w628) -> ("Cycle End Time"=w310:u32, "Cycles Run"=w308:u32, "Cycle Start Time"=w306:u32, "Starting Estimated Time"=w303:u16, "Starting Target Moisture"=w301:u16, "Starting Inlet Temp"=w299:u16, "Starting Outlet Temp"=w297:u16, "Max Inlet Temp"=w296:u16, "Max Outlet Temp"=w293:u16, "Actual Cycle Time"=w291:u16, "Raw Moisture After Target"=w289:u16, "Time To Target Voltage"=w287:u16, "DOD Temp Multiplier"=w285:u16, "DOD Multiplier"=w283:u8, "DOD Time Adder"=w281:u8, "Base Cycle Time Before\nTarget Voltage"=w279:u8, "Base Cycle Time After\nTarget Voltage"=w277:u8, "Internal Cycle ID"=w275:u8, "Restriction Detected"=w61:enum8{"Unknown", "Small", "Large"}, "Aggregated Load Size"=w59:enum8{"Unknown", "Small", "Large"}, "Load Size By Contact"=w57:enum8{"Unknown", "Small", "Large"}, "Load Size By Temperature"=w55:enum8{"Unknown", "Small", "Large"}, "Pause Key Press Count"=w273:u8, "Door Open Count"=w271:u8, "Door Latch Count"=w269:u8, "System Reset Count"=w267:u8, "Fault Occurred Flag"=w266:bool, "Delay Flag"=w263:bool, "My Cycle Flag"=w261:bool, "Blackout Flag"=w259:bool, "Fallback Heat Control\nInvoked Flag"=w257:bool, "Empty Drum \nDetected Flag"=w255:bool, "Dry Load \nDetected Flag"=w253:bool, "Drum Ground Watchdog\nDetected Flag"=w251:bool, "Cycle Started\nRemotely Flag"=w249:bool, "Extended Tumble\nStarted Remotely Flag"=w247:bool, "Cycle Cancelled\nRemotely Flag"=w245:bool, "Edry Option At Start"=w243:bool, "Edry Option At End"=w242:bool, "Damp Alert\nOption At Start"=w239:bool, "Damp Alert\nOption At End"=w237:bool, "Clean Lint Filter\nStatus At Start"=w235:bool, "Detangle Option\nAt Start"=w233:bool, "Detangle Option\nAt End"=w231:bool, "Control Lock\nOption At Start"=w229:bool, "Control Lock\nOption At End"=w226:bool, "Curvature Algorithm\nTripped"=w225:bool, "Over Temp\nOccurred Flag"=w221:bool, "Trimmer Algorithm\nTripped"=w220:bool, "Sense Mode Flag"=w219:bool, "Dryness Level At Start"=w53:T5, "Dryness Level At End"=w50:T5, "Temp Level At Start"=w49:T6, "Temp Level At End"=w47:T6, "Time Setting At Start"=w216:u8, "Time Setting At End"=w215:u8, "Alert Volume Level At Start"=w45:enum8{"Off", "Low", "Medium", "High"}, "Alert Volume Level At End"=w43:enum8{"Off", "Low", "Medium", "High"}, "Trimmer Trip Count\nHeater 1 & 2 Combined"=w213:u8, "Trimmer Trip Count\nHeater 1"=w201:u8, "Trimmer Trip Count\nHeater 2"=w71:u8, "EOC Reason"=w70:T7, "Cycle Selected"=w68:string, "Extended Tumble Option At Start"=w207:bool, "Extended Tumble Option At End"=w206:bool, "Drum Light Option At Start"=w205:bool, "Drum Light Option At End"=w204:bool, "Rack Dry Flag"=w203:bool, "My Settings Flag"=w64:bool, "Warm Up"=w62:bool, "Delay Minutes"=w67:u16, "Max Filtered Moisture\nVoltage (Sensed Cycle)"=w21:u16, "Final Target\nMoisture Voltage"=w20:u16)
  n342 = case shown="\"Event Sequence Communication Issue\"" w70 {
    tunnel: ["N/A" "EMPTY DRUM" "DRY LOAD" "COOL DOWN PAUSED" "EXTENDED TUMBLE PAUSED" "KNOB CHANGE" "POWER KEY" "NORMAL" "Event Sequence Communication Issue"] -> w69
    frame "N/A" {
    }
    frame "Empty Drum" {
    }
    frame "Dry Load" {
    }
    frame "Cool Down Paused" {
    }
    frame "Extended Tumble Paused" {
    }
    frame "Knob Change" {
    }
    frame "Power Key" {
    }
    frame "Normal" {
    }
    frame "Event Sequence Communication Issue" {
    }
  }
  n343 = case shown="False" w62 {
    tunnel: ["FALSE" "TRUE"] -> w63
    frame False {
    }
    frame True {
    }
  }
  n344 = case shown="False" w64 {
    tunnel: ["FALSE" "TRUE"] -> w65
    frame False {
    }
    frame True {
    }
  }
  n345 = case shown="False" w203 {
    tunnel: ["FALSE" "TRUE"] -> w208
    frame False {
    }
    frame True {
    }
  }
  n346 = case shown="False" w204 {
    tunnel: ["FALSE" "TRUE"] -> w209
    frame False {
    }
    frame True {
    }
  }
  n347 = case shown="False" w205 {
    tunnel: ["FALSE" "TRUE"] -> w210
    frame False {
    }
    frame True {
    }
  }
  n348 = Number To Decimal String(number=w20) -> (decimal integer string=w18:string)  [unwired: 1 in]
  n349 = Number To Decimal String(number=w21) -> (decimal integer string=w19:string)  [unwired: 1 in]
  n350 = case shown="\"Off\"" w43 {
    tunnel: ["OFF" "LOW" "MEDIUM" "HIGH"] -> w42
    frame "Off" {
    }
    frame "Low" {
    }
    frame "Medium" {
    }
    frame "High" {
    }
  }
  n351 = case shown="False" w206 {
    tunnel: ["FALSE" "TRUE"] -> w211
    frame False {
    }
    frame True {
    }
  }
  n352 = case shown="False" w207 {
    tunnel: ["FALSE" "TRUE"] -> w212
    frame False {
    }
    frame True {
    }
  }
  n353 = Number To Decimal String(number=w67) -> (decimal integer string=w66:string)  [unwired: 1 in]
  n354 = case shown="\"Off\"" w45 {
    tunnel: ["OFF" "LOW" "MEDIUM" "HIGH"] -> w44
    frame "Off" {
    }
    frame "Low" {
    }
    frame "Medium" {
    }
    frame "High" {
    }
  }
  n355 = case shown="\"No Heat\"" w47 {
    tunnel: ["NO HEAT" "EXTRA LOW" "LOW" "MEDIUM" "HIGH"] -> w46
    frame "No Heat" {
    }
    frame "Extra Low" {
    }
    frame "Low" {
    }
    frame "Medium" {
    }
    frame "High" {
    }
  }
  n356 = case shown="\"No Heat\"" w49 {
    tunnel: ["NO HEAT" "EXTRA LOW" "LOW" "MEDIUM" "HIGH"] -> w48
    frame "No Heat" {
    }
    frame "Extra Low" {
    }
    frame "Low" {
    }
    frame "Medium" {
    }
    frame "High" {
    }
  }
  n357 = case shown="\"Extra Dry\"" w50 {
    tunnel: ["DISABLED" "DAMP" "LESS DRY" "DRY" "MORE DRY" "EXTRA DRY"] -> w51
    frame "Disabled" {
    }
    frame "Damp" {
    }
    frame "Less Dry" {
    }
    frame "Dry" {
    }
    frame "More Dry" {
    }
    frame "Extra Dry" {
    }
  }
  n358 = case shown="\"Extra Dry\"" w53 {
    tunnel: ["DISABLED" "DAMP" "LESS DRY" "DRY" "MORE DRY" "EXTRA DRY"] -> w52
    frame "Disabled" {
    }
    frame "Damp" {
    }
    frame "Less Dry" {
    }
    frame "Dry" {
    }
    frame "More Dry" {
    }
    frame "Extra Dry" {
    }
  }
  n359 = Format Into String(w71) -> (resulting string=w72:string)  [unwired: 3 in, 1 out]
  n360 = Format Into String(w201) -> (resulting string=w202:string)  [unwired: 3 in, 1 out]
  n361 = case shown="False" w219 {
    tunnel: ["FALSE" "TRUE"] -> w222
    frame False {
    }
    frame True {
    }
  }
  n362 = Number To Decimal String(number=w213) -> (decimal integer string=w214:string)  [unwired: 1 in]
  n363 = case shown="False" w220 {
    tunnel: ["FALSE" "TRUE"] -> w223
    frame False {
    }
    frame True {
    }
  }
  n364 = case shown="False" w221 {
    tunnel: ["FALSE" "TRUE"] -> w224
    frame False {
    }
    frame True {
    }
  }
  n365 = case shown="False" w225 {
    tunnel: ["FALSE" "TRUE"] -> w227
    frame False {
    }
    frame True {
    }
  }
  n366 = case shown="False" w226 {
    tunnel: ["FALSE" "TRUE"] -> w228
    frame False {
    }
    frame True {
    }
  }
  n367 = Number To Decimal String(number=w215) -> (decimal integer string=w217:string)  [unwired: 1 in]
  n368 = Number To Decimal String(number=w216) -> (decimal integer string=w218:string)  [unwired: 1 in]
  n369 = case shown="False" w229 {
    tunnel: ["FALSE" "TRUE"] -> w230
    frame False {
    }
    frame True {
    }
  }
  n370 = case shown="False" w231 {
    tunnel: ["FALSE" "TRUE"] -> w232
    frame False {
    }
    frame True {
    }
  }
  n371 = case shown="False" w233 {
    tunnel: ["FALSE" "TRUE"] -> w234
    frame False {
    }
    frame True {
    }
  }
  n372 = case shown="False" w235 {
    tunnel: ["FALSE" "TRUE"] -> w236
    frame False {
    }
    frame True {
    }
  }
  n373 = case shown="False" w237 {
    tunnel: ["FALSE" "TRUE"] -> w238
    frame False {
    }
    frame True {
    }
  }
  n374 = case shown="False" w239 {
    tunnel: ["FALSE" "TRUE"] -> w240
    frame False {
    }
    frame True {
    }
  }
  n375 = case shown="False" w242 {
    tunnel: ["FALSE" "TRUE"] -> w241
    frame False {
    }
    frame True {
    }
  }
  n376 = case shown="False" w243 {
    tunnel: ["FALSE" "TRUE"] -> w244
    frame False {
    }
    frame True {
    }
  }
  n377 = case shown="False" w245 {
    tunnel: ["FALSE" "TRUE"] -> w246
    frame False {
    }
    frame True {
    }
  }
  n378 = case shown="False" w247 {
    tunnel: ["FALSE" "TRUE"] -> w248
    frame False {
    }
    frame True {
    }
  }
  n379 = case shown="False" w249 {
    tunnel: ["FALSE" "TRUE"] -> w250
    frame False {
    }
    frame True {
    }
  }
  n380 = case shown="False" w251 {
    tunnel: ["FALSE" "TRUE"] -> w252
    frame False {
    }
    frame True {
    }
  }
  n381 = case shown="False" w253 {
    tunnel: ["FALSE" "TRUE"] -> w254
    frame False {
    }
    frame True {
    }
  }
  n382 = case shown="False" w255 {
    tunnel: ["FALSE" "TRUE"] -> w256
    frame False {
    }
    frame True {
    }
  }
  n383 = case shown="False" w257 {
    tunnel: ["FALSE" "TRUE"] -> w258
    frame False {
    }
    frame True {
    }
  }
  n384 = case shown="False" w259 {
    tunnel: ["FALSE" "TRUE"] -> w260
    frame False {
    }
    frame True {
    }
  }
  n385 = case shown="False" w261 {
    tunnel: ["FALSE" "TRUE"] -> w262
    frame False {
    }
    frame True {
    }
  }
  n386 = case shown="False" w263 {
    tunnel: ["FALSE" "TRUE"] -> w264
    frame False {
    }
    frame True {
    }
  }
  n387 = case shown="False" w266 {
    tunnel: ["FALSE" "TRUE"] -> w265
    frame False {
    }
    frame True {
    }
  }
  n388 = case shown="\"Unknown\"" w55 {
    tunnel: ["UNKNOWN" "SMALL" "LARGE"] -> w54
    frame "Unknown" {
    }
    frame "Small" {
    }
    frame "Large" {
    }
  }
  n389 = case shown="\"Unknown\"" w57 {
    tunnel: ["UNKNOWN" "SMALL" "LARGE"] -> w56
    frame "Unknown" {
    }
    frame "Small" {
    }
    frame "Large" {
    }
  }
  n390 = case shown="\"Unknown\"" w59 {
    tunnel: ["UNKNOWN" "SMALL" "LARGE"] -> w58
    frame "Unknown" {
    }
    frame "Small" {
    }
    frame "Large" {
    }
  }
  n391 = case shown="\"Unknown\"" w61 {
    tunnel: ["UNKNOWN" "SMALL" "LARGE"] -> w60
    frame "Unknown" {
    }
    frame "Small" {
    }
    frame "Large" {
    }
  }
  n392 = Number To Decimal String(number=w267) -> (decimal integer string=w268:string)  [unwired: 1 in]
  n393 = Number To Decimal String(number=w269) -> (decimal integer string=w270:string)  [unwired: 1 in]
  n394 = Number To Decimal String(number=w271) -> (decimal integer string=w272:string)  [unwired: 1 in]
  n395 = Number To Decimal String(number=w273) -> (decimal integer string=w274:string)  [unwired: 1 in]
  n396 = Number To Decimal String(number=w275) -> (decimal integer string=w276:string)  [unwired: 1 in]
  n397 = Number To Decimal String(number=w277) -> (decimal integer string=w278:string)  [unwired: 1 in]
  n398 = Number To Decimal String(number=w279) -> (decimal integer string=w280:string)  [unwired: 1 in]
  n399 = Number To Decimal String(number=w281) -> (decimal integer string=w282:string)  [unwired: 1 in]
  n400 = Number To Decimal String(number=w283) -> (decimal integer string=w284:string)  [unwired: 1 in]
  n401 = Number To Decimal String(number=w285) -> (decimal integer string=w286:string)  [unwired: 1 in]
  n402 = Number To Decimal String(number=w287) -> (decimal integer string=w288:string)  [unwired: 1 in]
  n403 = Number To Decimal String(number=w289) -> (decimal integer string=w290:string)  [unwired: 1 in]
  n404 = Number To Decimal String(number=w291) -> (decimal integer string=w292:string)  [unwired: 1 in]
  n405 = Number To Decimal String(number=w293) -> (decimal integer string=w294:string)  [unwired: 1 in]
  n406 = Number To Decimal String(number=w296) -> (decimal integer string=w295:string)  [unwired: 1 in]
  n407 = Number To Decimal String(number=w297) -> (decimal integer string=w298:string)  [unwired: 1 in]
  n408 = Number To Decimal String(number=w299) -> (decimal integer string=w300:string)  [unwired: 1 in]
  n409 = Number To Decimal String(number=w301) -> (decimal integer string=w302:string)  [unwired: 1 in]
  n410 = Number To Decimal String(number=w303) -> (decimal integer string=w304:string)  [unwired: 1 in]
  n411 = Number To Decimal String(number=w306) -> (decimal integer string=w305:string)  [unwired: 1 in]
  n412 = Number To Decimal String(number=w308) -> (decimal integer string=w307:string)  [unwired: 1 in]
  n413 = Number To Decimal String(number=w310) -> (decimal integer string=w309:string)  [unwired: 1 in]
  n414 = Build Array(w309, w307, w305, w304, w302, w300, w298, w295, w294, w292, w290, w288, w286, w284, w282, w280, w278, w276, w60, w58, w56, w54, w274, w272, w270, w268, w265, w264, w262, w260, w258, w256, w254, w252, w250, w248, w246, w244, w241, w240, w238, w236, w234, w232, w230, w228, w227, w224, w223, w222, w52, w51, w48, w46, w218, w217, w44, w42, w214, w202, w72, w69, w68, w212, w211, w210, w209, w208, w65, w63, w66, w19, w18) -> (→"String Array Out":string[])
